vi "BuildServerROS.vi"(3 "Node ROS":T2={"topic port"=0, "Node"="", "topic"="", "type"="", "node port"=0, "error "={"status"=FALSE, "code"=0, "source"=""}, "Direction"=enum."Node", "APIs"=[], "Update (ms)"=1, "write queue"=1}, 4 "port":u16, 5 "New Subscriber":T4) -> (2 "data":T1={"New Subscriber"={"Caller ID"="", "Topic Name"="", "Protocol"="", "URIs"="", "ID"=refnum}, "ROS of Server"={"topic port"=0, "Node"="", "topic"="", "type"="", "node port"=0, "error "={"status"=FALSE, "code"=0, "source"=""}, "Direction"=enum."Node", "APIs"=[], "Update (ms)"=1, "write queue"=1}, "new port"=0})   [LabVIEW 2012]
uses:
  SubVIs/_ROSDirection.ctl
  SubVIs/_ROSControl.ctl
  requestTopic.ctl
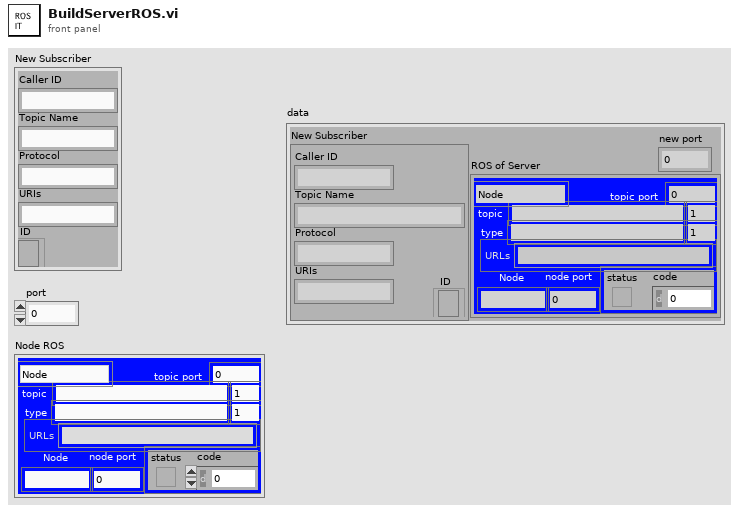
[diagram p1: front panel]
types:
  T1 = typedef "requestTopic.ctl" = cluster{"New Subscriber":cluster{"Caller ID":string, "Topic Name":string, "Protocol":string, "URIs":string, "ID":refnum<k5>}, "ROS of Server":T2, "new port":u16}
  T2 = typedef "_ROSControl.ctl" = cluster{"topic port":u16, "Node":string, "topic":string, "type":string, "node port":u32, "error ":errorcluster, "Direction":T3, "APIs":string[], "Update (ms)":u16, "write queue":u16}
  T3 = typedef "_ROSDirection.ctl" = enum16{"Node", "Publisher", "Subscriber", "Service Client"}
  T4 = cluster{"Caller ID":string, "Topic Name":string, "Protocol":string, "URIs":string, "ID":refnum<k5>}
  T5 = cluster{"New Subscriber":cluster{"Caller ID":string, "Topic Name":string, "Protocol":string, "URIs":string, "ID":refnum<k5>}, "Node ROS":T2, "port":u16}
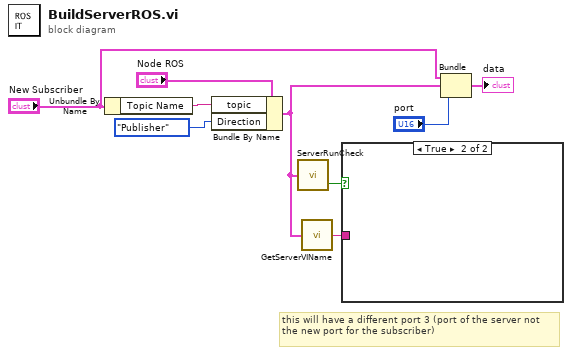
[diagram p0: block diagram]
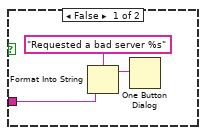
[diagram p2: hidden frame]
diagram:
  # "this will have a different port 3 (port of the server not the new port for the subscriber)"
  n1 = Unbundle By Name("New Subscriber") -> ("Topic Name"=w8:string)
  n2 = Bundle By Name(cluster="Node ROS", "topic"=w8, "Direction"=_ROSDirection."Publisher") -> (w2:T2)
  n3 = call "ServerRunCheck.vi"("ROS in"=w2) -> ("Running?"=w4:bool)  [unwired: 1 out]
  n4 = call "GetServerVIName.vi"("ROS"=w2) -> ("vi name"=w3:string)
  n5 = case shown="True" w4 {
    tunnel: w3 -> [w11 _]
    frame False {
      n6 = Format Into String(format string="Requested a bad server %s", w11) -> (resulting string=w10:string)  [unwired: 2 in, 1 out]
      n7 = One Button Dialog(message=w10) -> ()  [unwired: 1 in, 1 out]
    }
    frame True {
    }
  }
  n8 = Bundle("New Subscriber"="New Subscriber", "Node ROS"=w2, "port"="port") -> (→"data":T5)  [unwired: 1 in]
